vi "BinarizationRegistration.vi"(8 "error in":errorcluster, 9 "Binarization parameters":T1={"threshold percentage"=95.0, "equalize?"=FALSE, "Method (clustering)"=0} {"Method (clustering)" items=["clustering", "entropy", "metric", "moments", "inter-class variance"]}, 10 "Roy":T2, 11 "Rob":T2) -> (0 "error out":errorcluster, 1 "quality":dbl, 2 "y translation":dbl, 3 "x translation":dbl)   [LabVIEW 2012]
uses:
  <vilib>/vision/Image Controls.llb/IMAQ Image.ctl
  BinarizationParameters.ctl
  <vilib>/gmath/statdist.llb/st_Percentiles (scalar).vi
  <vilib>/vision/NI_Vision_Development_Module.lvlib
  <vilib>/gmath/NI_Gmath.lvlib
panel:
  out "bin roy":T2(plugin-control)
  out "bin rob":T2(plugin-control)
  out "bin cc":T2(plugin-control)
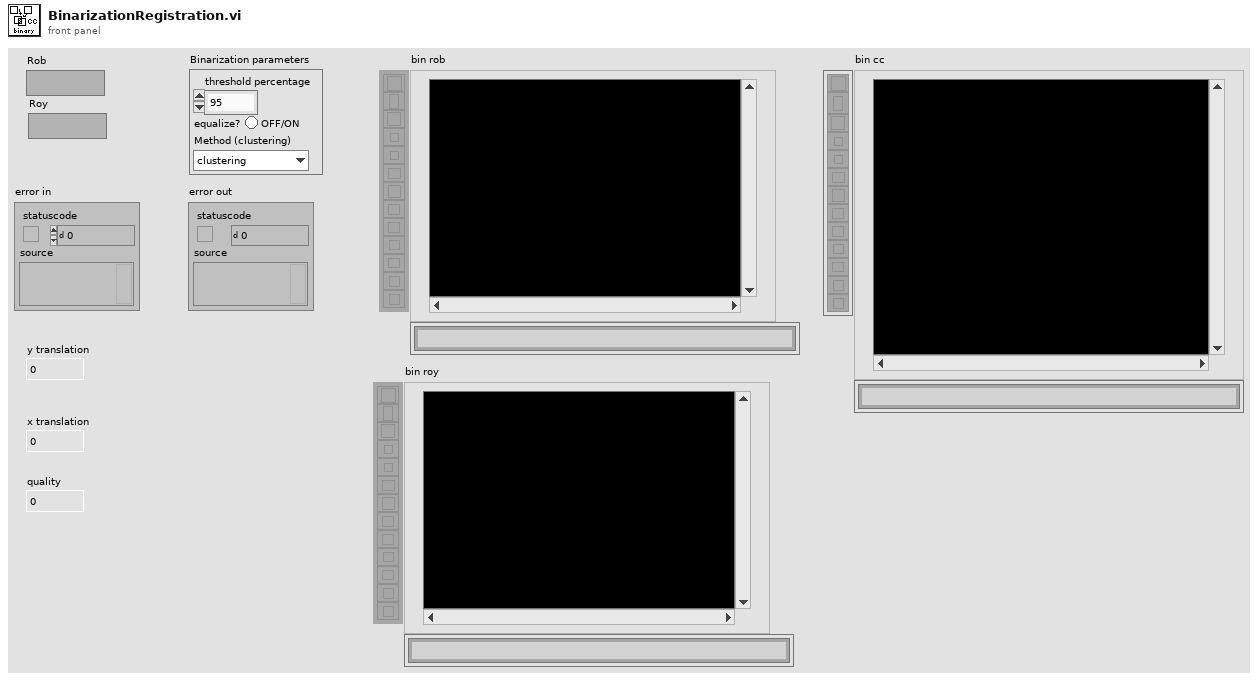
[diagram p1: front panel]
types:
  T1 = typedef "BinarizationParameters.ctl" = cluster{"threshold percentage":dbl, "equalize?":bool, "Method (clustering)":i32}
  T2 = typedef "IMAQ Image.ctl" = refnum<image>
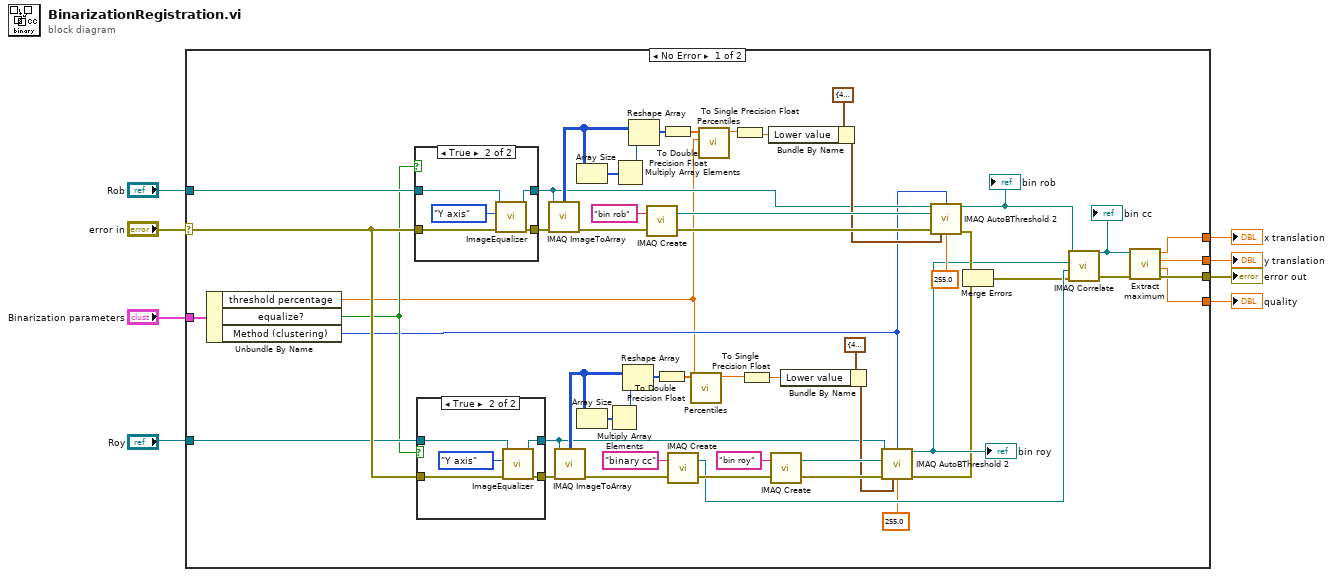
[diagram p0: block diagram]
diagram:
  n1 = case shown="No Error" "error in" {
    selector: "error in" -> [w23 w76]
    tunnel: [w15 _] -> w8
    tunnel: [w13 _] -> w7
    tunnel: [w16 w76] -> w6
    tunnel: "Rob" -> [w26 _]
    tunnel: "Roy" -> [w22 _]
    tunnel: [w14 _] -> w2
    tunnel: "Binarization parameters" -> [w12 _]
    frame No Error {
      n2 = Unbundle By Name(w12) -> ("threshold percentage"=w9:dbl, "equalize?"=w11:bool, "Method (clustering)"=w10:i32)
      n3 = case shown="True" w11 {
        tunnel: [w69 w75] -> w27
        tunnel: w26 -> [w70 w74]
        tunnel: [w70 w73] -> w25
        tunnel: w23 -> [w69 w71]
        frame False {
        }
        frame True {
          n4 = call "ImageEqualizer.vi"("error in (no error)"=w71, "axis to equalize"=enum16{"X axis", "Y axis"}."Y axis", "Image in"=w74) -> ("error out"=w75:errorcluster, "Image out"=w73:T2)  [unwired: 7 in]
        }
      }
      n5 = case shown="True" w11 {
        tunnel: [w62 w68] -> w24
        tunnel: w23 -> [w62 w67]
        tunnel: w22 -> [w63 w65]
        tunnel: [w63 w64] -> w21
        frame False {
        }
        frame True {
          n6 = call "ImageEqualizer.vi"("error in (no error)"=w67, "axis to equalize"=enum16{"X axis", "Y axis"}."Y axis", "Image in"=w65) -> ("error out"=w68:errorcluster, "Image out"=w64:T2)  [unwired: 7 in]
        }
      }
      n7 = call "IMAQ ImageToArray"("error in (no error)"=w27, "Image"=w25) -> ("error out"=w35:errorcluster, "Image Pixels (U8)"=w42:u8[][])  [unwired: 2 in, 3 out]
      n8 = call "IMAQ ImageToArray"("error in (no error)"=w24, "Image"=w21) -> ("error out"=w20:errorcluster, "Image Pixels (U8)"=w34:u8[][])  [unwired: 2 in, 3 out]
      n9 = Array Size(array=w42) -> (size(s)=w40:i32[])
      n10 = Array Size(array=w34) -> (size(s)=w32:i32[])
      n11 = Multiply Array Elements(1:w32) -> (0:w33:i32)
      n12 = Multiply Array Elements(1:w40) -> (0:w41:i32)
      n13 = Reshape Array(w34, w33) -> (w31:u8[])
      n14 = Reshape Array(w42, w41) -> (w39:u8[])
      n15 = call "IMAQ Create"("Image Name"="bin rob", "error in (no error)"=w35) -> ("New Image"=w57:T2, "error out"=w58:errorcluster)  [unwired: 3 in]
      n16 = To Double Precision Float(number=w31) -> (double precision float=w30:dbl[])
      n17 = To Double Precision Float(number=w39) -> (double precision float=w38:dbl[])
      n18 = call "IMAQ Create"("Image Name"="binary cc", "error in (no error)"=w20) -> ("New Image"=w53:T2, "error out"=w54:errorcluster)  [unwired: 3 in]
      n19 = call-poly <vilib>:"Percentiles.vi"("p"=w9, "x array"=w30) -> ("percentile"=w29:dbl)  [unwired: 8 in, 1 out]
      n20 = call-poly <vilib>:"Percentiles.vi"("p"=w9, "x array"=w38) -> ("percentile"=w37:dbl)  [unwired: 8 in, 1 out]
      n21 = To Single Precision Float(number=w37) -> (single precision float=w36:sgl)
      n22 = To Single Precision Float(number=w29) -> (single precision float=w28:sgl)
      n23 = Bundle By Name(cluster=cluster{"Lower value":sgl, "Upper value":sgl} {"Lower value"=40.0, "Upper value"=255.0} ("Threshold Limits"), "Lower value"=w36) -> (w45:cluster{"Lower value":sgl, "Upper value":sgl})
      n24 = call "IMAQ Create"("Image Name"="bin roy", "error in (no error)"=w54) -> ("New Image"=w56:T2, "error out"=w55:errorcluster)  [unwired: 3 in]
      n25 = Bundle By Name(cluster=cluster{"Lower value":sgl, "Upper value":sgl} {"Lower value"=40.0, "Upper value"=255.0} ("Threshold Limits"), "Lower value"=w28) -> (w43:cluster{"Lower value":sgl, "Upper value":sgl})
      n26 = call "IMAQ AutoBThreshold 2"("Image Src"=w21, "Method (clustering)"=w10, "Image Dst"=w56, "error in (no error)"=w55, "Threshold Limits"=w43, "Replace Value (1)"=sgl 255.0) -> ("Image Dst Out"=w49:T2, "error out"=w48:errorcluster)  [unwired: 7 in, 1 out]
      "bin roy" <- w49
      n27 = call "IMAQ AutoBThreshold 2"("Image Src"=w25, "Method (clustering)"=w10, "Image Dst"=w57, "error in (no error)"=w58, "Threshold Limits"=w45, "Replace Value (1)"=sgl 255.0) -> ("Image Dst Out"=w51:T2, "error out"=w50:errorcluster)  [unwired: 7 in, 1 out]
      "bin rob" <- w51
      n28 = Merge Errors(w50, w48) -> (w18:errorcluster)
      n29 = call "IMAQ Correlate"("Image Src"=w51, "Image Template"=w49, "Image Dst"=w53, "error in (no error)"=w18) -> ("Image Dst Out"=w17:T2, "error out"=w19:errorcluster)  [unwired: 3 in]
      "bin cc" <- w17
      n30 = call "Extract maximum.vi"("error in (no error)"=w19, "Image in"=w17) -> ("error out"=w16:errorcluster, "Max value"=w13:dbl, "y translation"=w14:dbl, "x translation"=w15:dbl)  [unwired: 6 in]
    }
    frame Error {
    }
  }
  "error out" <- w6
  "x translation" <- w8
  "quality" <- w7
  "y translation" <- w2
